vi "SignalToNode(viaString).vi"(0 "Tree DVR in":refnum<data-value>, 1 "NodePath":string, 2 "y-axis (Data Range)":dbl[](array[numeric]), 3 "Start Time":dbl, 4 "Delta t":dbl, 5 "error in (no error)":errorcluster) -> (6 "Tree DVR out":refnum<data-value>, 7 "TreeNode DVR out":refnum<data-value>, 8 "Error Message Output":errorcluster)   [LabVIEW 2013]
uses:
  <vilib>/MDSplus/Classes/Data_Class/TreeNode_Class/TreeNode.lvclass
  <vilib>/MDSplus/Classes/Tree_Class/Tree.lvclass
  <vilib>/MDSplus/Classes/Data_Class/Compound_Class/Signal_Class/Signal.lvclass
  <vilib>/MDSplus/Library/MDSplus.lvlib
panel:
  out "error out 2":errorcluster
  out "Signal DVR out":refnum<data-value>
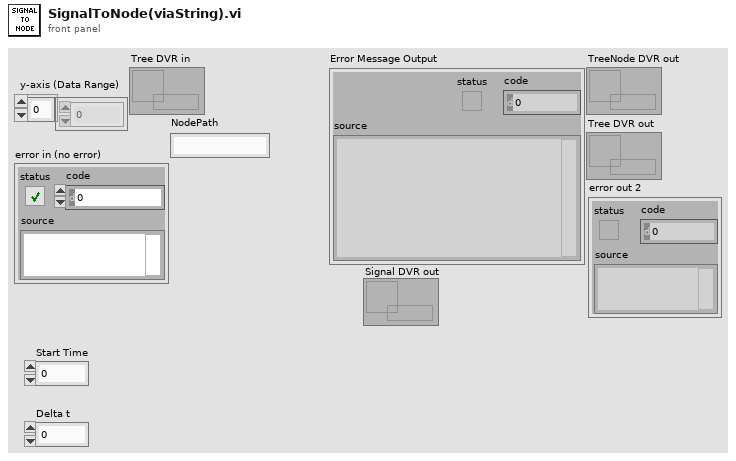
[diagram p1: front panel]
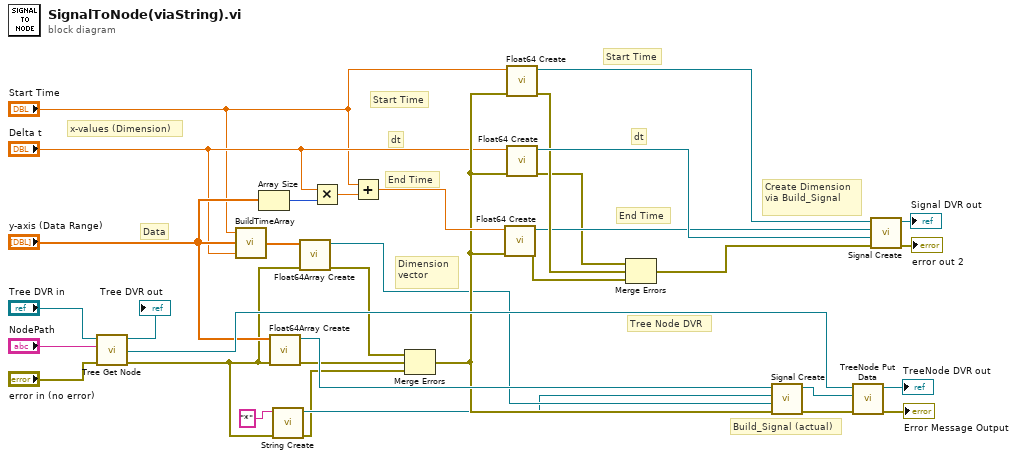
[diagram p0: block diagram]
diagram:
  # "Build_Signal (actual)"
  # "Create Dimension via Build_Signal"
  # "Dimension vector"
  # "x-values (Dimension)"
  # "Tree Node DVR"
  # "Data"
  # "dt"
  # "End Time"
  # "Start Time"
  # "Start Time"
  # "dt"
  # "End Time"
  n1 = call <vilib>:"Tree Get Node.vi"("error in (no error)"="error in (no error)", "Path"="NodePath", "Tree DVR in"="Tree DVR in") -> ("error out"=w1:errorcluster, "Node out"=w22:refnum<data-value>, "Tree DVR out"=→"Tree DVR out":refnum<data-value>)  [unwired: 6 in]
  n2 = call "BuildTimeArray.vi"("Time Increment (dt)"="Delta t", "Data Array (y-values)"="y-axis (Data Range)", "Start Time (t_o)"="Start Time") -> ("Time Array (x-values)"=w7:dbl[])
  n3 = Array Size(array="y-axis (Data Range)") -> (size(s)=w11:i32)
  n4 = call <vilib>:"Float64Array Create.vi"("error in (no error)"=w1, "DBL array in"="y-axis (Data Range)") -> ("error out"=w16:errorcluster, "Float64Array DVR out"=w17:refnum<data-value>)  [unwired: 8 in]
  n5 = call <vilib>:"String Create.vi"("error in (no error)"=w1, "String value in"="*") -> ("error out"=w2:errorcluster, "String DVR out"=w3:refnum<data-value>)  [unwired: 8 in]
  n6 = call <vilib>:"Float64Array Create.vi"("error in (no error)"=w1, "DBL array in"=w7) -> ("error out"=w6:errorcluster, "Float64Array DVR out"=w5:refnum<data-value>)  [unwired: 8 in]
  n7 = Multiply(x="Delta t", y=w11) -> (x*y=w30:dbl)
  n8 = Add(x="Start Time", y=w30) -> (x+y=w24:dbl)
  n9 = Merge Errors(w6, w16, w2) -> (w14:errorcluster)
  n10 = call <vilib>:"Float64 Create.vi"("error in (no error)"=w14, "DBL in"=w24) -> ("error out"=w25:errorcluster, "Float64 DVR out"=w23:refnum<data-value>)  [unwired: 8 in]
  n11 = call <vilib>:"Float64 Create.vi"("error in (no error)"=w14, "DBL in"="Start Time") -> ("error out"=w27:errorcluster, "Float64 DVR out"=w26:refnum<data-value>)  [unwired: 8 in]
  n12 = call <vilib>:"Float64 Create.vi"("error in (no error)"=w14, "DBL in"="Delta t") -> ("error out"=w19:errorcluster, "Float64 DVR out"=w28:refnum<data-value>)  [unwired: 8 in]
  n13 = Merge Errors(w19, w27, w25) -> (w29:errorcluster)
  n14 = call <vilib>:"Signal Create.vi"("error in (no error)"=w14, "Dimension"=w5, "Raw"=w3, "Data"=w17) -> ("error out"=w18:errorcluster, "Signal DVR out"=w15:refnum<data-value>)  [unwired: 6 in]
  n15 = call <vilib>:"TreeNode Put Data.vi"("error in (no error)"=w18, "Data"=w15, "TreeNode DVR in"=w22) -> ("error out"=→"Error Message Output":errorcluster, "TreeNode DVR out"=→"TreeNode DVR out":refnum<data-value>)  [unwired: 7 in]
  n16 = call <vilib>:"Signal Create.vi"("error in (no error)"=w29, "Dimension"=w28, "Raw"=w23, "Data"=w26) -> ("error out"=→"error out 2":errorcluster, "Signal DVR out"=→"Signal DVR out":refnum<data-value>)  [unwired: 6 in]
